vi "YFM.vi"() -> ()   [LabVIEW 2017]
uses:
  <vilib>/Analysis/6fits.llb/Curve Fitting Criteria.ctl
  <vilib>/DAQmx/write.llb/DAQmx Write (Analog DBL 1Chan 1Samp).vi
  <vilib>/DAQmx/read.llb/DAQmx Read (Analog Wfm 1Chan NSamp).vi
  <vilib>/DAQmx/create/channels.llb/DAQmx Create Channel (AO-Voltage-Basic).vi
  <vilib>/DAQmx/create/channels.llb/DAQmx Create Channel (AI-Voltage-Basic).vi
  <vilib>/DAQmx/configure/timing.llb/DAQmx Timing (Sample Clock).vi
  <vilib>/DAQmx/miscellaneous.llb/DAQmx Fill In Error Info.vi
  <vilib>/Analysis/6fits.llb/1D B-Spline Fit.vi
  <vilib>/Analysis/NI_AALPro.lvlib
panel:
  out "Gm":dbl=1.2807365889988531
  out "XY Graph":cluster{dbl[], dbl[]}[](graph)=[{[1.0, 1.01, 1.02, 1.03, 1.04, 1.05, 1.06, 1.07, 1.08, 1.09, 1.1, 1.11, 1.12, 1.13, 1.1400000000000001, 1.15, 1.16, 1.17, 1.18, 1.19, 1.2, 1.21, 1.22, 1.23, 1.24, 1.25, 1.26, 1.27, 1.28, 1.29, 1.3, 1.31, 1.32, 1.33, 1.34, 1.35, 1.3599999999999999, 1.37, 1.38, 1.3900000000000001, 1.4, 1.4100000000000001, 1.42, 1.43, 1.44, 1.45, 1.46, 1.47, 1.48, 1.49, 1.5, 1.51, 1.52, 1.53, 1.54, 1.55, 1.56, 1.57, 1.58, 1.5899999999999999, 1.6, 1.6099999999999999, 1.62, 1.63, 1.6400000000000001, 1.65, 1.6600000000000001, 1.67, 1.6800000000000002, 1.69, 1.7000000000000002, 1.71, 1.72, 1.73, 1.74, 1.75, 1.76, 1.77, 1.78, 1.79, 1.8], [0.0001406837966681925, 0.00017329260568865743, 0.00020820674483461386, 0.0002473363178110047, 0.00029259156888969244, 0.00034588268704838936, 0.0004091199374159651, 0.00048421339254229516, 0.0005730740394266775, 0.0006776123997716339, 0.0007997395001033244, 0.0009413670035303315, 0.0011044157276307017, 0.0012908291709391622, 0.0015025449661566722, 0.0017415038658703606, 0.002009635851919069, 0.0023089080255293635, 0.0026412573650695216, 0.00300862715765009, 0.003412928394349637, 0.00385619455965326, 0.0043403422192649956, 0.004866982619634445, 0.0054354544559452895, 0.0060446058777508, 0.0066930000320852764, 0.007379242394393755, 0.008101713962559164, 0.008859512321748893, 0.00965106438500263, 0.010474966566325053, 0.011329470154085093, 0.01221395555673069, 0.013126663262881937, 0.014066256748937257, 0.015031339825726471, 0.016019996159249948, 0.01703208644671035, 0.018065602172593308, 0.019119286944481645, 0.02019094630523743, 0.02128076665309128, 0.022386685619805495, 0.02350724466378253, 0.024640191239451662, 0.025785831977718974, 0.02694036462873089, 0.02810016214549338, 0.029260622976395277, 0.03041992169179588, 0.03157352666580087, 0.03271759327527242, 0.03384778038006183, 0.03496212349447369, 0.036056019613731324, 0.037125833309573274, 0.03816722686474849, 0.03917838986449462, 0.04015688173229741, 0.04110096409918942, 0.042009018990437776, 0.042879048350750175, 0.043710279653658195, 0.044500657951924295, 0.04524860464035054, 0.04595230870865961, 0.04661059131746005, 0.047221637131112854, 0.047784015114188755, 0.04829927306434063, 0.04877172701719982, 0.04920549046942062, 0.04960477949228663, 0.04997376300697568, 0.05031671196216749, 0.05063778958006266, 0.05094118974875579, 0.05123109590890491, 0.05151172994453984, 0.05178726874445318]}, {[1.0, 1.01, 1.02, 1.03, 1.04, 1.05, 1.06, 1.07, 1.08, 1.09, 1.1, 1.11, 1.12, 1.13, 1.1400000000000001, 1.15, 1.16, 1.17, 1.18, 1.19, 1.2, 1.21, 1.22, 1.23, 1.24, 1.25, 1.26, 1.27, 1.28, 1.29, 1.3, 1.31, 1.32, 1.33, 1.34, 1.35, 1.3599999999999999, 1.37, 1.38, 1.3900000000000001, 1.4, 1.4100000000000001, 1.42, 1.43, 1.44, 1.45, 1.46, 1.47, 1.48, 1.49, 1.5, 1.51, 1.52, 1.53, 1.54, 1.55, 1.56, 1.57, 1.58, 1.5899999999999999, 1.6, 1.6099999999999999, 1.62, 1.63, 1.6400000000000001, 1.65, 1.6600000000000001, 1.67, 1.6800000000000002, 1.69, 1.7000000000000002, 1.71, 1.72, 1.73, 1.74, 1.75, 1.76, 1.77, 1.78, 1.79, 1.8], [0.00034195886629488035, 0.002627125847793829, 0.003828147634465611, 0.004479552479574878, 0.005053409303142192, 0.005868254267166494, 0.0069315855811519, 0.008219592067563055, 0.009709533493506858, 0.01136380211120237, 0.013179441897194513, 0.015154687785685031, 0.017337747530183995, 0.01976964024003242, 0.022394621071960333, 0.025198340340269305, 0.02827270430828352, 0.03168317692612576, 0.035196296736626734, 0.03879716842613748, 0.042665075023935545, 0.04683889269637367, 0.050835358444763265, 0.05464454015133892, 0.05850825839088328, 0.06264801341314526, 0.06641014489183081, 0.06995365760524827, 0.0735209348589122, 0.0774051005974433, 0.08079850916275924, 0.08399961875310634, 0.08706011099321807, 0.09022550308470895, 0.0928542809721528, 0.09531536196458515, 0.09769975312126349, 0.09996189607224716, 0.10244552670653367, 0.10455950960303886, 0.10662674228097889, 0.10846002568004821, 0.11033727461597292, 0.11172283235356574, 0.112961204211051, 0.11385095417347352, 0.11456341250094391, 0.11493214055627331, 0.11505633439568709, 0.11492822095904956, 0.11453579896096897, 0.11397268218172701, 0.11310593703455347, 0.11212059642738566, 0.11076571666734532, 0.10913978925975704, 0.10679001615737056, 0.10422015258326718, 0.1011764365748735, 0.09776360150836928, 0.09391732503002838, 0.08915151481199372, 0.08473657504703438, 0.0803526821116575, 0.07566861835517767, 0.07051485926488872, 0.06597188729296785, 0.06179840921133788, 0.057625436537780704, 0.0534014920479649, 0.049771630022713065, 0.04651155016939106, 0.04337799174867856, 0.04025456000907884, 0.037303234464824635, 0.03434180233449164, 0.0312103706279972, 0.028323290804630835, 0.026512210941898116, 0.02631061274913672, 0.028390034101172336]}]
  in  "average point":dbl=100.0
  out "intercept":dbl=-0.8504234856344423
  in  "Ring":dbl(ring)=1000.0 items=["1uA/V"=1000000.0, "10uA/V"=100000.0, "50uA/V"=50000.0, "100uA/V"=10000.0, "1mA/V"=1000.0]
  out "theta avg.":dbl=5.368752441146047
  in  "stop_theta":dbl=1.7
  in  "start_theta":dbl=1.65
  out "theta":dbl[](array[numeric])=[4.94931298731623, 5.180216295642689, 4.825285093633401, 5.0929475430887265, 5.937033050907736, 6.2277196762875064]
  in  "theta0":dbl
  out "Rct":dbl=4.1919255585122155
  out "YFM":dbl[](array[numeric])=[0.08821215663779128, 0.092082568962766, 0.09907016920127037, 0.10234880530465468, 0.10321969159971099, 0.10759200588404398, 0.11559672512341536, 0.12040160799131543, 0.12146984104373643, 0.12661381449616713, 0.13274273225748492, 0.14365722351142726, 0.15018894616529568, 0.1522697579899892, 0.15981375750488686, 0.17298044297697612, 0.18153431900574607, 0.1839604877740676, 0.19324171931041195, 0.20946261745466693, 0.21941871069919475]
  out "Vg":dbl[](array[numeric])=[1.5, 1.51, 1.52, 1.53, 1.54, 1.55, 1.56, 1.57, 1.58, 1.5899999999999999, 1.6, 1.6099999999999999, 1.62, 1.63, 1.6400000000000001, 1.65, 1.6600000000000001, 1.67, 1.6800000000000002, 1.69, 1.7000000000000002]
  in  "stop_linear":dbl=1.7
  in  "start_linear":dbl=1.5
  out "(Gm*Vd)^1/2":dbl=0.6198556095573032
  out "Vt":dbl=1.3719702984406466
  out "theta":cluster{dbl[], dbl[]}(graph)={[1.0, 1.01, 1.02, 1.03, 1.04, 1.05, 1.06, 1.07, 1.08, 1.09, 1.1, 1.11, 1.12, 1.13, 1.1400000000000001, 1.15, 1.16, 1.17, 1.18, 1.19, 1.2, 1.21, 1.22, 1.23, 1.24, 1.25, 1.26, 1.27, 1.28, 1.29, 1.3, 1.31, 1.32, 1.33, 1.34, 1.35, 1.3599999999999999, 1.37, 1.38, 1.3900000000000001, 1.4, 1.4100000000000001, 1.42, 1.43, 1.44, 1.45, 1.46, 1.47, 1.48, 1.49, 1.5, 1.51, 1.52, 1.53, 1.54, 1.55, 1.56, 1.57, 1.58, 1.5899999999999999, 1.6, 1.6099999999999999, 1.62, 1.63, 1.6400000000000001, 1.65, 1.6600000000000001, 1.67, 1.6800000000000002, 1.69, 1.7000000000000002, 1.71, 1.72, 1.73, 1.74, 1.75, 1.76, 1.77, 1.78, 1.79, 1.8], [8.773271295930094, 3.1794245406011132, 3.318850587282279, 3.423220821044215, 3.515962700547965, 3.646843875313869, 3.8329685242913363, 3.9755451837460236, 4.105730579917826, 4.283551156712209, 4.483065921442678, 4.771353235894191, 4.99747482088341, 5.211102602597867, 5.518527959614132, 5.959926362175338, 6.325258661637671, 6.669395876358629, 7.183832987227901, 7.937294922458045, 8.586326570087659, 9.23284804522201, 10.190474899722048, 11.642478017219997, 13.062830567250689, 14.473676158760725, 16.666947867825222, 20.296257146334586, 24.251846973252725, 28.730688837820672, 36.330830932663844, 49.99412924006109, 68.97002482428867, 98.78190784877637, 165.9442159322073, 343.2166460662854, 1201.9545005147454, 42960.269209324186, 2378.4201019031148, 460.84075148053483, 200.8159646646415, 106.43491609269758, 60.050460907557586, 40.33358864241725, 31.9670575559515, 23.890075855374086, 16.836172615027312, 13.50381108757487, 12.391485346289269, 10.35024792105223, 7.813957347449366, 6.852103076058092, 6.92801333487301, 6.098909679754331, 4.858453901498248, 4.516682005572691, 4.854525452439907, 4.650668134169877, 3.9002243260113243, 3.8052751180395212, 3.84541511950552, 4.44866172511922, 4.517182152660376, 4.086041332018803, 4.251024918178202, 4.94931298731623, 5.180216295642689, 4.825285093633401, 5.0929475430887265, 5.937033050907736, 6.2277196762875064, 5.940018058789697, 6.285785489104267, 7.2177304094683485, 7.628393925763401, 7.285799617143395, 7.716374155469511, 8.880100550973964, 9.366333033675646, 9.07134155413153, 7.480646195738274]}
  out "YFM":cluster{dbl[], "Best Linear Fit":dbl[]}(graph)={[1.5, 1.51, 1.52, 1.53, 1.54, 1.55, 1.56, 1.57, 1.58, 1.5899999999999999, 1.6, 1.6099999999999999, 1.62, 1.63, 1.6400000000000001, 1.65, 1.6600000000000001, 1.67, 1.6800000000000002, 1.69, 1.7000000000000002], "Best Linear Fit"=[0.07935992870151265, 0.08555848479708561, 0.09175704089265868, 0.09795559698823175, 0.10415415308380471, 0.11035270917937778, 0.11655126527495085, 0.12274982137052382, 0.1289483774660969, 0.13514693356166985, 0.14134548965724292, 0.14754404575281588, 0.15374260184838906, 0.1599411579439619, 0.1661397140395352, 0.17233827013510805, 0.17853682623068112, 0.1847353823262542, 0.19093393842182727, 0.19713249451740011, 0.2033310506129734]}
  out "gm":cluster{dbl[], dbl[]}(graph)={[1.0, 1.01, 1.02, 1.03, 1.04, 1.05, 1.06, 1.07, 1.08, 1.09, 1.1, 1.11, 1.12, 1.13, 1.1400000000000001, 1.15, 1.16, 1.17, 1.18, 1.19, 1.2, 1.21, 1.22, 1.23, 1.24, 1.25, 1.26, 1.27, 1.28, 1.29, 1.3, 1.31, 1.32, 1.33, 1.34, 1.35, 1.3599999999999999, 1.37, 1.38, 1.3900000000000001, 1.4, 1.4100000000000001, 1.42, 1.43, 1.44, 1.45, 1.46, 1.47, 1.48, 1.49, 1.5, 1.51, 1.52, 1.53, 1.54, 1.55, 1.56, 1.57, 1.58, 1.5899999999999999, 1.6, 1.6099999999999999, 1.62, 1.63, 1.6400000000000001, 1.65, 1.6600000000000001, 1.67, 1.6800000000000002, 1.69, 1.7000000000000002, 1.71, 1.72, 1.73, 1.74, 1.75, 1.76, 1.77, 1.78, 1.79, 1.8], [0.00034195886629488035, 0.002627125847793829, 0.003828147634465611, 0.004479552479574878, 0.005053409303142192, 0.005868254267166494, 0.0069315855811519, 0.008219592067563055, 0.009709533493506858, 0.01136380211120237, 0.013179441897194513, 0.015154687785685031, 0.017337747530183995, 0.01976964024003242, 0.022394621071960333, 0.025198340340269305, 0.02827270430828352, 0.03168317692612576, 0.035196296736626734, 0.03879716842613748, 0.042665075023935545, 0.04683889269637367, 0.050835358444763265, 0.05464454015133892, 0.05850825839088328, 0.06264801341314526, 0.06641014489183081, 0.06995365760524827, 0.0735209348589122, 0.0774051005974433, 0.08079850916275924, 0.08399961875310634, 0.08706011099321807, 0.09022550308470895, 0.0928542809721528, 0.09531536196458515, 0.09769975312126349, 0.09996189607224716, 0.10244552670653367, 0.10455950960303886, 0.10662674228097889, 0.10846002568004821, 0.11033727461597292, 0.11172283235356574, 0.112961204211051, 0.11385095417347352, 0.11456341250094391, 0.11493214055627331, 0.11505633439568709, 0.11492822095904956, 0.11453579896096897, 0.11397268218172701, 0.11310593703455347, 0.11212059642738566, 0.11076571666734532, 0.10913978925975704, 0.10679001615737056, 0.10422015258326718, 0.1011764365748735, 0.09776360150836928, 0.09391732503002838, 0.08915151481199372, 0.08473657504703438, 0.0803526821116575, 0.07566861835517767, 0.07051485926488872, 0.06597188729296785, 0.06179840921133788, 0.057625436537780704, 0.0534014920479649, 0.049771630022713065, 0.04651155016939106, 0.04337799174867856, 0.04025456000907884, 0.037303234464824635, 0.03434180233449164, 0.0312103706279972, 0.028323290804630835, 0.026512210941898116, 0.02631061274913672, 0.028390034101172336]}
  out "Id Array":dbl[](array[numeric])=[0.00014380519924163819, 0.00017251508998870847, 0.0002069907772541046, 0.00024246901950836184, 0.00029009391360282913, 0.0003470001416206361, 0.0004138472720623018, 0.0004825208067893985, 0.0005732423384666444, 0.0006800900890350343, 0.0008053428339481357, 0.0009501924426078798, 0.0010955655836105342, 0.001285666178226471, 0.0015028227405548102, 0.0017481948445320125, 0.0019905994954109198, 0.0022993595335006737, 0.002646737241840363, 0.003026758996725083, 0.0033953897148609156, 0.0038553083641529105, 0.004356241488885881, 0.0049002408452987695, 0.005413576268577574, 0.006033570078611376, 0.0067062392254352565, 0.007416456315422052, 0.008066195990514755, 0.008842022349834442, 0.00965827844524383, 0.010504185347127916, 0.01127402047152519, 0.012182970369720467, 0.0131194410680294, 0.014089293952608118, 0.015080395623254772, 0.015971339051914214, 0.01701860930485725, 0.018080461238336565, 0.019173157799005518, 0.0201442702067375, 0.021271933876800538, 0.02242474280862809, 0.0235855412434101, 0.024608846741914773, 0.02578779699435233, 0.02696931771883965, 0.028155614788293832, 0.029198198753070847, 0.03038262245087622, 0.03157079385528559, 0.032733587359428405, 0.03375418423786163, 0.03490888993239402, 0.03604176775784494, 0.03715319636774064, 0.038107772435045234, 0.039156711134719836, 0.04018605925683977, 0.04117144947133066, 0.04211004037003515, 0.04288993695836065, 0.04374108134493827, 0.04454030844278336, 0.045294570088577284, 0.04591159516110419, 0.04657382554898262, 0.04719352635331153, 0.04776669541873929, 0.04823360777149202, 0.048733151610755886, 0.04919220434637067, 0.04961998226437567, 0.04996556118321418, 0.050333132079029085, 0.05067486940593717, 0.0509870598399639, 0.05123985956754684, 0.05150794522676469, 0.05175410695796015]
  out "Vg Array":dbl[](array[numeric])=[1.0, 1.01, 1.02, 1.03, 1.04, 1.05, 1.06, 1.07, 1.08, 1.09, 1.1, 1.11, 1.12, 1.13, 1.1400000000000001, 1.15, 1.16, 1.17, 1.18, 1.19, 1.2, 1.21, 1.22, 1.23, 1.24, 1.25, 1.26, 1.27, 1.28, 1.29, 1.3, 1.31, 1.32, 1.33, 1.34, 1.35, 1.3599999999999999, 1.37, 1.38, 1.3900000000000001, 1.4, 1.4100000000000001, 1.42, 1.43, 1.44, 1.45, 1.46, 1.47, 1.48, 1.49, 1.5, 1.51, 1.52, 1.53, 1.54, 1.55, 1.56, 1.57, 1.58, 1.5899999999999999, 1.6, 1.6099999999999999, 1.62, 1.63, 1.6400000000000001, 1.65, 1.6600000000000001, 1.67, 1.6800000000000002, 1.69, 1.7000000000000002, 1.71, 1.72, 1.73, 1.74, 1.75, 1.76, 1.77, 1.78, 1.79, 1.8]
  out "transfer characteristic":cluster{dbl[], dbl[]}(graph)={[1.0, 1.01, 1.02, 1.03, 1.04, 1.05, 1.06, 1.07, 1.08, 1.09, 1.1, 1.11, 1.12, 1.13, 1.1400000000000001, 1.15, 1.16, 1.17, 1.18, 1.19, 1.2, 1.21, 1.22, 1.23, 1.24, 1.25, 1.26, 1.27, 1.28, 1.29, 1.3, 1.31, 1.32, 1.33, 1.34, 1.35, 1.3599999999999999, 1.37, 1.38, 1.3900000000000001, 1.4, 1.4100000000000001, 1.42, 1.43, 1.44, 1.45, 1.46, 1.47, 1.48, 1.49, 1.5, 1.51, 1.52, 1.53, 1.54, 1.55, 1.56, 1.57, 1.58, 1.5899999999999999, 1.6, 1.6099999999999999, 1.62, 1.63, 1.6400000000000001, 1.65, 1.6600000000000001, 1.67, 1.6800000000000002, 1.69, 1.7000000000000002, 1.71, 1.72, 1.73, 1.74, 1.75, 1.76, 1.77, 1.78, 1.79, 1.8], [0.0001406837966681925, 0.00017329260568865743, 0.00020820674483461386, 0.0002473363178110047, 0.00029259156888969244, 0.00034588268704838936, 0.0004091199374159651, 0.00048421339254229516, 0.0005730740394266775, 0.0006776123997716339, 0.0007997395001033244, 0.0009413670035303315, 0.0011044157276307017, 0.0012908291709391622, 0.0015025449661566722, 0.0017415038658703606, 0.002009635851919069, 0.0023089080255293635, 0.0026412573650695216, 0.00300862715765009, 0.003412928394349637, 0.00385619455965326, 0.0043403422192649956, 0.004866982619634445, 0.0054354544559452895, 0.0060446058777508, 0.0066930000320852764, 0.007379242394393755, 0.008101713962559164, 0.008859512321748893, 0.00965106438500263, 0.010474966566325053, 0.011329470154085093, 0.01221395555673069, 0.013126663262881937, 0.014066256748937257, 0.015031339825726471, 0.016019996159249948, 0.01703208644671035, 0.018065602172593308, 0.019119286944481645, 0.02019094630523743, 0.02128076665309128, 0.022386685619805495, 0.02350724466378253, 0.024640191239451662, 0.025785831977718974, 0.02694036462873089, 0.02810016214549338, 0.029260622976395277, 0.03041992169179588, 0.03157352666580087, 0.03271759327527242, 0.03384778038006183, 0.03496212349447369, 0.036056019613731324, 0.037125833309573274, 0.03816722686474849, 0.03917838986449462, 0.04015688173229741, 0.04110096409918942, 0.042009018990437776, 0.042879048350750175, 0.043710279653658195, 0.044500657951924295, 0.04524860464035054, 0.04595230870865961, 0.04661059131746005, 0.047221637131112854, 0.047784015114188755, 0.04829927306434063, 0.04877172701719982, 0.04920549046942062, 0.04960477949228663, 0.04997376300697568, 0.05031671196216749, 0.05063778958006266, 0.05094118974875579, 0.05123109590890491, 0.05151172994453984, 0.05178726874445318]}
  in  "Vd":dbl=0.3
  in  "Vd channels":tag="Dev3/ao1"
  in  "Id channels":tag="Dev9/ai0"
  out "# of step":dbl=81.0
  in  "Step":dbl=0.01
  in  "Stop (V)":dbl=1.8
  in  "Start (V)":dbl=1.0
  in  "Vg channels":tag="Dev3/ao0"
  # "<theta range>"
  # "<linear region>"
  # "Vg"
  # "Fitting"
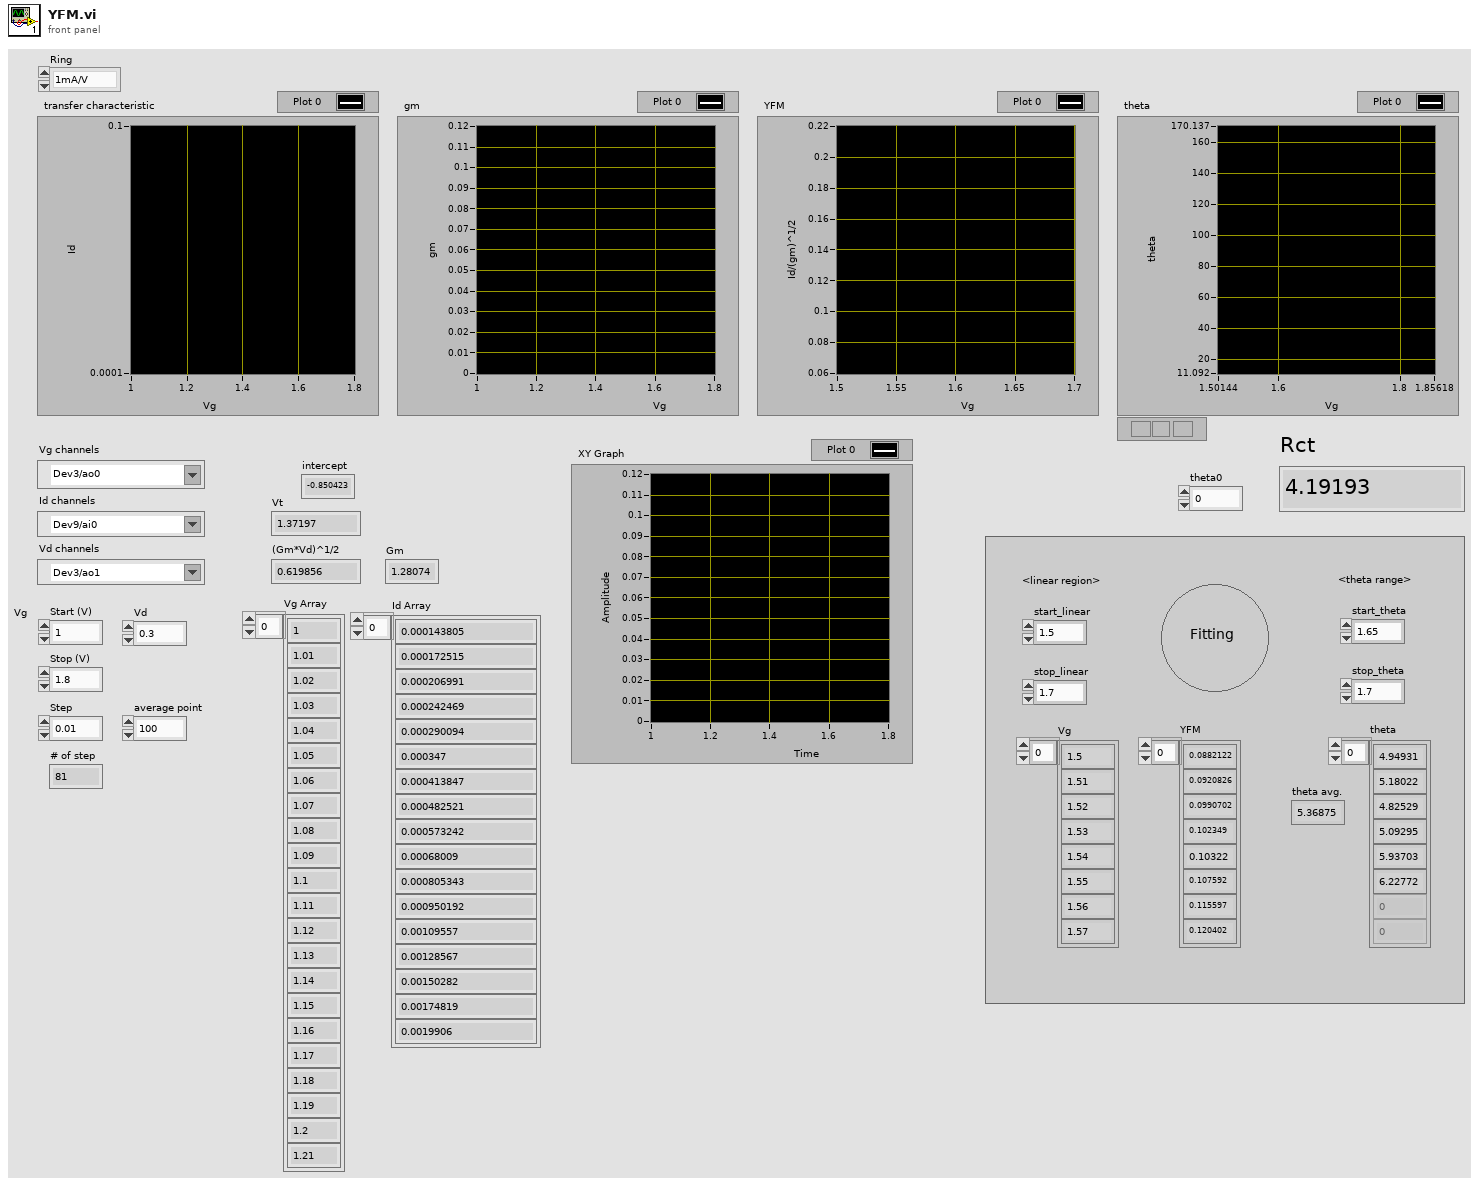
[diagram p1: front panel]
types:
  T1 = typedef "NI_AALPro.lvlib/Curve Fitting Criteria.ctl" = u16
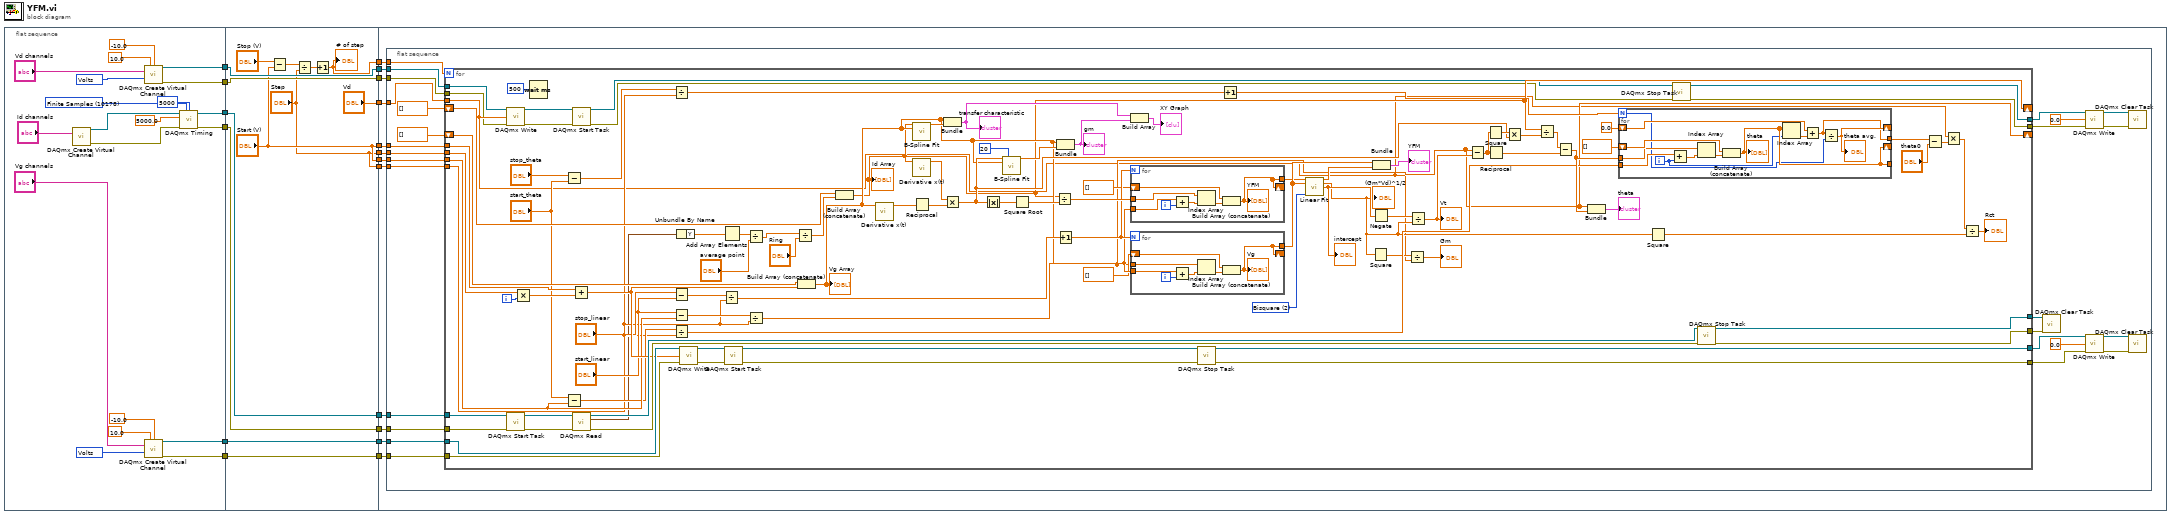
[diagram p0: block diagram]
diagram:
  n1 = flat-sequence {
    tunnel: [w28] -> w6
    tunnel: [w27] -> w5
    tunnel: [w34] -> w2
    tunnel: [w33] -> w1
    tunnel: [w21] -> w4
    tunnel: [w20] -> w3
    tunnel: w6 -> [w51]
    tunnel: w5 -> [w50]
    tunnel: w4 -> [w49]
    tunnel: w3 -> [w48]
    tunnel: [w51] -> w18
    tunnel: [w50] -> w17
    tunnel: [w49] -> w16
    tunnel: [w48] -> w15
    tunnel: ["Step"] -> w14
    tunnel: ["Start (V)"] -> w13
    tunnel: ["Vd"] -> w12
    tunnel: [w44] -> w11
    tunnel: w2 -> [w44]
    tunnel: [w43] -> w10
    tunnel: w1 -> [w43]
    tunnel: [w41] -> w9
    tunnel: ["Start (V)"] -> w8
    tunnel: ["Step"] -> w7
    tunnel: w18 -> [w61]
    tunnel: w17 -> [w60]
    tunnel: w16 -> [w59]
    tunnel: w15 -> [w58]
    tunnel: w14 -> [w63]
    tunnel: w13 -> [w62]
    tunnel: w12 -> [w57]
    tunnel: w11 -> [w53]
    tunnel: w10 -> [w52]
    tunnel: w9 -> [w56]
    tunnel: w8 -> [w55]
    tunnel: w7 -> [w54]
    frame #0 {
      w23 = 10178 items=["Finite Samples"=10178, "Continuous Samples"=10123, "Hardware Timed Single Point"=12522] ("sample mode")
      w29 = 10348 items=["Volts"=10348, "From Custom Scale"=10065] ("units")
      w35 = 10348 items=["Volts"=10348, "From Custom Scale"=10065] ("units")
      n2 = call-poly <vilib>:"DAQmx Create Virtual Channel.vi"("physical channels"="Id channels") -> ("task out"=w25:refnum<k21>, "error out"=w24:errorcluster)  [unwired: 13 in]
      n3 = call-poly <vilib>:"DAQmx Create Virtual Channel.vi"("maximum value"=10.0, "minimum value"=-10.0, "physical channels"="Vd channels", "units"=w35) -> ("task out"=w34:refnum<k21>, "error out"=w33:errorcluster)  [unwired: 10 in]
      n4 = call-poly <vilib>:"DAQmx Create Virtual Channel.vi"("maximum value"=10.0, "minimum value"=-10.0, "physical channels"="Vg channels", "units"=w29) -> ("task out"=w28:refnum<k21>, "error out"=w27:errorcluster)  [unwired: 10 in]
      n5 = call-poly <vilib>:"DAQmx Timing.vi"("task/channels in"=w25, "sample mode"=w23, "samples per channel"=5000, "rate"=5000.0, "error in"=w24) -> ("task out"=w21:refnum<k21>, "error out"=w20:errorcluster)  [unwired: 9 in]
    }
    frame #1 {
      n6 = Subtract(x="Stop (V)", y="Start (V)") -> (x-y=w47:dbl)
      n7 = Divide(x=w47, y="Step") -> (x/y=w42:dbl)
      n8 = Increment(x=w42) -> (x+1=w41:dbl)
      "# of step" <- w41
    }
    frame #2 {
      n9 = flat-sequence {
        tunnel: w63 -> [w88]
        tunnel: w62 -> [w89]
        tunnel: w57 -> [w79]
        tunnel: w56 -> [w87]
        tunnel: w59 -> [w86]
        tunnel: w58 -> [w85]
        tunnel: w61 -> [w84]
        tunnel: w60 -> [w83]
        tunnel: w55 -> [w81]
        tunnel: w54 -> [w80]
        tunnel: w53 -> [w67]
        tunnel: w52 -> [w66]
        frame #0 {
          n10 = for {
            N: w87 -> [_]
            tunnel: w89 -> [w187]
            tunnel: w88 -> [w186]
            tunnel: w86 -> [w184]
            tunnel: w85 -> [w185]
            tunnel: w84 -> [w179]
            tunnel: w83 -> [w178]
            shift-right: [w112] -> _
            shift-left: dbl[] [] -> [w172]
            shift-right: [w111] -> _
            shift-left: dbl[] [] -> [w171]
            tunnel: w81 -> [w129]
            tunnel: w80 -> [w127]
            tunnel: w79 -> [w94]
            tunnel: [w104] -> w72
            tunnel: [w103] -> w70
            tunnel: [w102] -> w69
            tunnel: [w101] -> w68
            tunnel: w67 -> [w95]
            tunnel: w66 -> [w93]
            tunnel: [w92] -> w65
            tunnel: [w91] -> w64
            i -> [w173]
            w149 = T1 2 items=["Least Square", "Least Absolute Residual", "Bisquare"] ("method")
            n11 = call-poly <vilib>:"DAQmx Write.vi"("task/channels in"=w95, "data"=w94, "error in"=w93) -> ("task out"=w96:refnum<k21>, "error out"=w98:errorcluster)  [unwired: 10 in, 1 out]
            n12 = call <vilib>:"DAQmx Start Task.vi"("task/channels in"=w184, "error in"=w185) -> ("task out"=w183:refnum<k21>, "error out"=w182:errorcluster)  [unwired: 12 in]
            n13 = Multiply(x=w186, y=w173) -> (x*y=w188:dbl)
            n14 = Wait (ms)(milliseconds to wait=u32 500) -> ()  [unwired: 1 out]
            n15 = Subtract(x="stop_theta", y="start_theta") -> (x-y=w142:dbl)
            n16 = Subtract(x="start_theta", y=w129) -> (x-y=w128:dbl)
            n17 = call <vilib>:"DAQmx Start Task.vi"("task/channels in"=w96, "error in"=w98) -> ("task out"=w97:refnum<k21>, "error out"=w99:errorcluster)  [unwired: 12 in]
            n18 = Add(x=w187, y=w188) -> (x+y=w166:dbl)
            n19 = call-poly <vilib>:"DAQmx Read.vi"("task/channels in"=w183, "error in"=w182) -> ("task out"=w180:refnum<k21>, "data"=w123:waveform(dbl), "error out"=w181:errorcluster)  [unwired: 11 in]
            n20 = Divide(x=w142, y=w127) -> (x/y=w141:dbl)
            n21 = Subtract(x="stop_linear", y="start_linear") -> (x-y=w160:dbl)
            n22 = Subtract(x="start_linear", y=w129) -> (x-y=w157:dbl)
            n23 = Divide(x=w128, y=w127) -> (x/y=w126:dbl)
            n24 = Unbundle By Name(w123) -> ("Y"=w105:dbl[])
            n25 = call-poly <vilib>:"DAQmx Write.vi"("task/channels in"=w179, "data"=w166, "error in"=w178) -> ("task out"=w177:refnum<k21>, "error out"=w176:errorcluster)  [unwired: 10 in, 1 out]
            n26 = Divide(x=w160, y=w127) -> (x/y=w159:dbl)
            n27 = Add Array Elements(numeric array=w105) -> (sum=w122:dbl)
            n28 = call <vilib>:"DAQmx Start Task.vi"("task/channels in"=w177, "error in"=w176) -> ("task out"=w175:refnum<k21>, "error out"=w174:errorcluster)  [unwired: 12 in]
            n29 = Divide(x=w122, y="average point") -> (x/y=w121:dbl)
            n30 = Divide(x=w157, y=w127) -> (x/y=w150:dbl)
            n31 = Divide(x=w121, y="Ring") -> (x/y=w125:dbl)
            n32 = Build Array (concatenate)(w172, w166) -> (w112:dbl[])
            "Vg Array" <- w112
            n33 = Build Array (concatenate)(w171, w125) -> (w111:dbl[])
            "Id Array" <- w111
            n34 = call <vilib>:"Derivative x(t).vi"("X"=w112) -> ("dX/dt"=w169:dbl[])  [unwired: 9 in, 1 out]
            n35 = call-poly <vilib>:"B-Spline Fit.vi"("Y"=w111, "X"=w112) -> ("Best BSpline Fit Y"=w113:dbl[])  [unwired: 10 in, 3 out]
            n36 = call <vilib>:"Derivative x(t).vi"("X"=w111) -> ("dX/dt"=w170:dbl[])  [unwired: 9 in, 1 out]
            n37 = Reciprocal(x=w169) -> (1/x=w168:dbl[])
            n38 = Bundle(w112, "Best BSpline Fit Y"=w113) -> (w114:cluster{dbl[], "Best BSpline Fit Y":dbl[]})  [unwired: 1 in]
            "transfer characteristic" <- w114
            n39 = Multiply(x=w170, y=w168) -> (x*y=w116:dbl[])
            n40 = Absolute Value(x=w116) -> (abs(x)=w100:dbl[])
            n41 = call-poly <vilib>:"B-Spline Fit.vi"("Y"=w116, "# of control points"=20, "X"=w112) -> ("Best BSpline Fit Y"=w117:dbl[])  [unwired: 9 in, 3 out]
            n42 = Square Root(x=w100) -> (sqrt(x)=w167:dbl[])
            n43 = Divide(x=w111, y=w167) -> (x/y=w152:dbl[])
            n44 = Bundle(w112, "Best BSpline Fit Y"=w117) -> (w119:cluster{dbl[], "Best BSpline Fit Y":dbl[]})  [unwired: 1 in]
            "gm" <- w119
            n45 = Increment(x=w159) -> (x+1=w151:dbl)
            n46 = Build Array(w114, w119) -> (→"XY Graph":cluster{dbl[], "Best BSpline Fit Y":dbl[]}[])
            n47 = for {
              N: w151 -> [_]
              shift-right: [w202] -> _
              shift-left: dbl[] [] -> [w204]
              tunnel: w152 -> [w203]
              tunnel: [w202] -> w153
              tunnel: w150 -> [w201]
              i -> [w206]
              n48 = Add(x=w201, y=w206) -> (x+y=w207:dbl)
              n49 = Index Array(array=w203, index=w207) -> (element=w205:dbl)
              n50 = Build Array (concatenate)(w204, w205) -> (w202:dbl[])
              "YFM" <- w202
            }
            n51 = for {
              N: w151 -> [_]
              shift-right: [w209] -> _
              shift-left: dbl[] [] -> [w211]
              tunnel: w112 -> [w210]
              tunnel: [w209] -> w154
              tunnel: w150 -> [w208]
              i -> [w213]
              n52 = Add(x=w208, y=w213) -> (x+y=w214:dbl)
              n53 = Index Array(array=w210, index=w214) -> (element=w212:dbl)
              n54 = Build Array (concatenate)(w211, w212) -> (w209:dbl[])
              "Vg" <- w209
            }
            n55 = call <vilib>:"DAQmx Stop Task.vi"("task/channels in"=w175, "error in"=w174) -> ("task out"=w104:refnum<k21>, "error out"=w103:errorcluster)  [unwired: 12 in]
            n56 = Increment(x=w141) -> (x+1=w136:dbl)
            n57 = call <vilib>:"Linear Fit.vi"("Y"=w153, "X"=w154, "method"=w149) -> ("Best Linear Fit"=w156:dbl[], "slope"=w106:dbl, "intercept"=w133:dbl)  [unwired: 8 in, 2 out]
            "(Gm*Vd)^1/2" <- w106
            "intercept" <- w133
            n58 = Square(x=w106) -> (x^2=w108:dbl)
            n59 = Negate(x=w133) -> (-x=w132:dbl)
            n60 = Bundle(w154, "Best Linear Fit"=w156) -> (→"YFM":cluster{dbl[], "Best Linear Fit":dbl[]})  [unwired: 1 in]
            n61 = Divide(x=w108, y=w94) -> (x/y=→"Gm":dbl)
            n62 = Divide(x=w132, y=w106) -> (x/y=w131:dbl)
            "Vt" <- w131
            n63 = Subtract(x=w112, y=w131) -> (x-y=w165:dbl[])
            n64 = Square(x=w165) -> (x^2=w164:dbl[])
            n65 = Reciprocal(x=w165) -> (1/x=w145:dbl[])
            n66 = Multiply(x=w164, y=w116) -> (x*y=w163:dbl[])
            n67 = Divide(x=w111, y=w163) -> (x/y=w146:dbl[])
            n68 = Subtract(x=w146, y=w145) -> (x-y=w140:dbl[])
            n69 = Bundle(w112, w140) -> (→"theta":cluster{dbl[], dbl[]})  [unwired: 1 in]
            n70 = for {
              N: w136 -> [w191]
              shift-right: [w195] -> _
              shift-left: dbl[] [] -> [w198]
              tunnel: w140 -> [w197]
              tunnel: [w195] -> _
              tunnel: w126 -> [w196]
              shift-right: [w190] -> _
              shift-left: 0.0 -> [w193]
              tunnel: [w189] -> w138
              i -> [w194]
              n71 = Add(x=w196, y=w194) -> (x+y=w200:dbl)
              n72 = Index Array(array=w197, index=w200) -> (element=w199:dbl)
              n73 = Build Array (concatenate)(w198, w199) -> (w195:dbl[])
              "theta" <- w195
              n74 = Index Array(array=w195, index=w194) -> (element=w192:dbl)
              n75 = Add(x=w193, y=w192) -> (x+y=w190:dbl)
              n76 = Divide(x=w190, y=w191) -> (x/y=w189:dbl)
              "theta avg." <- w189
            }
            n77 = Square(x=w106) -> (x^2=w134:dbl)
            n78 = call <vilib>:"DAQmx Stop Task.vi"("task/channels in"=w97, "error in"=w99) -> ("task out"=w92:refnum<k21>, "error out"=w91:errorcluster)  [unwired: 12 in]
            n79 = call <vilib>:"DAQmx Stop Task.vi"("task/channels in"=w180, "error in"=w181) -> ("task out"=w102:refnum<k21>, "error out"=w101:errorcluster)  [unwired: 12 in]
            n80 = Subtract(x=w138, y="theta0") -> (x-y=w109:dbl)
            n81 = Multiply(x=w94, y=w109) -> (x*y=w110:dbl)
            n82 = Divide(x=w110, y=w134) -> (x/y=→"Rct":dbl)
          }
          n83 = call <vilib>:"DAQmx Clear Task.vi"("task in"=w69, "error in"=w68) -> ()  [unwired: 13 in, 1 out]
          n84 = call-poly <vilib>:"DAQmx Write.vi"("task/channels in"=w65, "data"=0.0, "error in"=w64) -> ("task out"=w76:refnum<k21>, "error out"=w77:errorcluster)  [unwired: 10 in, 1 out]
          n85 = call-poly <vilib>:"DAQmx Write.vi"("task/channels in"=w72, "data"=0.0, "error in"=w70) -> ("task out"=w73:refnum<k21>, "error out"=w74:errorcluster)  [unwired: 10 in, 1 out]
          n86 = call <vilib>:"DAQmx Clear Task.vi"("task in"=w76, "error in"=w77) -> ()  [unwired: 13 in, 1 out]
          n87 = call <vilib>:"DAQmx Clear Task.vi"("task in"=w73, "error in"=w74) -> ()  [unwired: 13 in, 1 out]
        }
      }
    }
  }
